vi "programa 11.vi"() -> ()   [LabVIEW 2011]
uses:
  <vilib>/express/express arith-compare/Formula/XNode/ExpressFormulaBlockNode.xnode
panel:
  out "Menor":dbl
  out "Mayor":dbl
  out "Promedio":dbl
  out "Contador":dbl
  out "NumeroPar":dbl
  # "Elaborar un programa donde se generen y presenten 5\nnumeros pares."
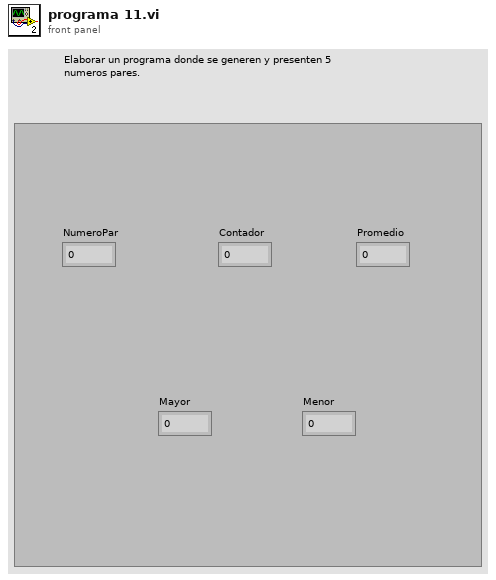
[diagram p1: front panel]
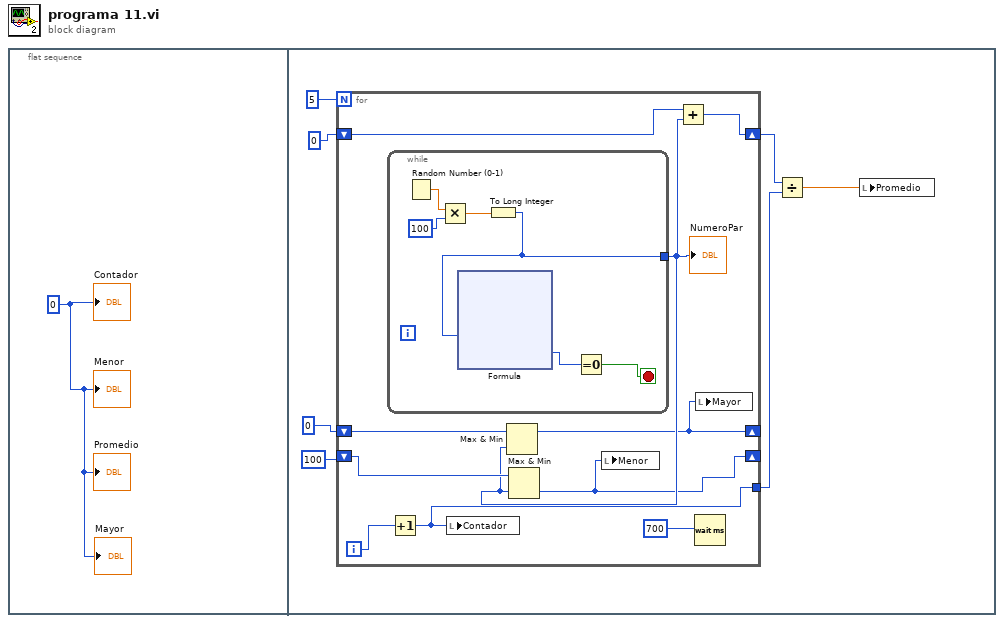
[diagram p0: block diagram]
diagram:
  n1 = flat-sequence {
    frame #0 {
      w1 = 0
      "Contador" <- w1
      "Mayor" <- w1
      "Menor" <- w1
      "Promedio" <- w1
    }
    frame #1 {
      n2 = for {
        N: 5 -> [_]
        shift-right: [w15] -> w6
        shift-left: 0 -> [w16]
        tunnel: [w13] -> w5
        shift-right: [w9] -> _
        shift-left: 0 -> [w14]
        shift-right: [w10] -> _
        shift-left: 100 -> [w12]
        i -> [w18]
        n3 = while {
          tunnel: [w19] -> w11
          stop <- w20 stop-if-true
          n4 = Random Number (0-1)() -> (number: 0 to 1=w23:dbl)
          n5 = Multiply(x=w23, y=100) -> (x*y=w24:dbl)
          n6 = To Long Integer(number=w24) -> (32bit integer=w19:i32)
          n7 = xnode "Formula"("X1"=w19) -> ("Result"=w21:i32)  [unwired: 1 in, 1 out]
          n8 = Equal To 0?(x=w21) -> (x = 0?=w20:bool)
        }
        "NumeroPar" <- w11
        n9 = Increment(x=w18) -> (x+1=w13:i32)
        n10 = local write "Contador"(w13) -> ()
        n11 = Max & Min(x=w14, y=w11) -> (max(x,y)=w9:i32)  [unwired: 1 out]
        n12 = Max & Min(x=w12, y=w11) -> (min(x,y)=w10:i32)  [unwired: 1 out]
        n13 = local write "Menor"(w10) -> ()
        n14 = Add(x=w16, y=w11) -> (x+y=w15:i32)
        n15 = Wait (ms)(milliseconds to wait=700) -> ()  [unwired: 1 out]
        n16 = local write "Mayor"(w9) -> ()
      }
      n17 = Divide(x=w6, y=w5) -> (x/y=w4:dbl)
      n18 = local write "Promedio"(w4) -> ()
    }
  }
